vi "FrozenFraction_Calcualte.vi"(8 "FreezeIdx":i32[](array[numeric])=[255, 322, 264, 271, 213, 293, 124, 126, 128, 125, 124, 129, 98, 99, 102, 99, 98, 98, 0, 81, 76, 73, 80, 73, 242, 225, 335, 285, 302, 293, 131, 126, 127, 130, 129, 126, 100, 105, 106, 99, 98, 99, 0, 73, 75, 79, 77, 71, 272, 219, 231, 224, 285, 293, 130, 135, 124, 133, 126, 135, 98, 99, 108, 99, 99, 98, 0, 76, 75, 0, 77, 76, 236, 192, 232, 228, 284, 240, 125, 125, 126, 137, 128, 126, 105, 106, 96, 110, 99, 100, 71, 80, 77, 79, 74, 77, 335, 254, 302, 233, 271, 287, 128, 133, 136, 127, 128, 133, 99, 107, 100, 108, 101, 101, 80, 77, 76, 74, 73, 74, 287, 301, 265, 290, 280, 272, 128, 136, 130, 124, 123, 130, 102, 99, 108, 100, 107, 100, 76, 76, 82, 75, 73, 74, 303, 321, 285, 279, 243, 273, 126, 126, 125, 126, 132, 124, 98, 108, 104, 111, 99, 106, 84, 76, 75, 82, 89, 72, 320, 283, 291, 240, 297, 236, 129, 131, 129, 124, 131, 126, 100, 105, 99, 100, 99, 101, 81, 81, 75, 76, 77, 75, 243, 307, 301, 286, 267, 129, 124, 132, 125, 127, 125, 124, 97, 104, 100, 99, 100, 100, 0, 88, 76, 73, 75, 75, 209, 309, 219, 296, 262, 217, 127, 131, 134, 127, 127, 124, 104, 100, 108, 107, 98, 99, 0, 77, 83, 80, 71, 76, 191, 248, 312, 218, 143, 278, 126, 126, 131, 133, 125, 126, 97, 100, 98, 99, 104, 100, 0, 78, 81, 75, 76, 75, 311, 257, 192, 162, 147, 252, 126, 126, 126, 130, 124, 123, 98, 98, 97, 98, 98, 99, 74, 79, 72, 73, 74, 73, 316, 253, 172, 122, 302, 135, 129, 129, 130, 124, 136, 125, 99, 103, 97, 101, 98, 98, 77, 74, 74, 82, 74, 77, 234, 193, 182, 305, 170, 153, 126, 132, 125, 133, 126, 125, 99, 98, 99, 99, 99, 102, 72, 74, 73, 73, 74, 73, 271, 240, 181, 300, 248, 288, 124, 125, 133, 132, 129, 124, 97, 97, 98, 99, 99, 99, 78, 81, 74, 75, 75, 73, 238, 259, 221, 128, 214, 192, 128, 128, 128, 124, 126, 129, 99, 99, 98, 99, 98, 98, 75, 78, 74, 79, 73, 75], 9 "Temps":dbl[][](graph)=array384x528[202752 elements], 10 "FreezeTemps":dbl[](array[numeric])=[-17.28714285714284, -23.360476190476163, -18.044761904761884, -18.98333333333329, -13.286190476190427, -20.920476190476165, -5.292380952380938, -5.350476190476172, -5.453809523809525, -5.195714285714246, -5.249047619047587, -5.483333333333292, -2.8057142857142594, -2.902380952380952, -2.915714285714273, -2.8785714285713766, -2.9642857142857224, -3.019999999999982, 0.0, -1.2985714285713925, -0.7119047619047478, -0.5214285714285438, -0.0428571428570876, -0.5152380952380895, -16.166190476190422, -14.609999999999957, -25.292857142857116, -20.543333333333294, -22.113333333333287, -21.32571428571424, -5.505238095238042, -5.593809523809512, -5.405714285714225, -5.401428571428539, -5.500952380952356, -5.363333333333287, -3.08095238095234, -3.0838095238095207, -3.0514285714285734, -3.015714285714239, -2.96333333333331, -3.152380952380952, 0.0, -0.61761904761903, -0.7347619047618537, -0.5952380952380736, -0.6928571428571217, -0.4047619047618696, -19.03666666666666, -14.313333333333276, -15.039047619047608, -14.185238095238049, -20.61285714285711, -21.26190476190473, -5.579523809523778, -5.624285714285691, -5.4423809523809155, -5.434761904761899, -5.471904761904739, -5.935238095238049, -3.0038095238095366, -2.935714285714255, -2.964761904761872, -3.1223809523809223, -3.133333333333269, -2.9828571428570854, 0.0, -1.0409523809523193, -0.8623809523809314, 0.0, -0.1014285714285847, -0.7966666666666242, -15.671428571428578, -11.62428571428569, -15.217142857142846, -14.780476190476179, -20.487619047619006, -16.03047619047618, -5.399523809523771, -5.3642857142857, -5.5033333333332735, -5.954285714285675, -5.610476190476163, -5.480476190476168, -3.2566666666666606, -3.0785714285713652, -2.83428571428567, -3.031904761904741, -3.0571428571428214, -3.1619047619047365, -0.6461904761904407, -1.014285714285677, -0.8404761904761813, -0.9290476190475943, -0.8390476190476193, -0.8742857142856906, -25.16952380952378, -17.619999999999976, -22.054285714285697, -14.887142857142862, -19.3942857142857, -20.490952380952336, -5.6619047619047365, -5.628571428571377, -5.825714285714241, -5.541904761904732, -5.704761904761881, -5.809523809523796, -3.402380952380952, -3.1676190476190413, -3.2052380952380872, -3.1780952380951817, -3.08428571428567, -3.1638095238095048, -1.1566666666666379, -0.8852380952380372, -0.9509523809523444, -0.784761904761865, -0.6295238095237892, -0.5247619047618741, -20.52047619047616, -22.020952380952338, -18.561428571428564, -21.041904761904732, -20.22999999999996, -19.46857142857138, -5.632380952380913, -5.829047619047628, -5.757619047619016, -5.409999999999968, -5.2971428571428305, -5.7942857142857065, -3.439047619047585, -3.210476190476129, -3.2157142857142276, -3.1152380952380554, -3.0599999999999454, -2.903809523809514, -0.9961904761904066, -1.029047619047617, -0.9152380952380668, -0.8190476190475806, -0.4390476190475852, -0.7114285714285415, -21.997619047619025, -23.774285714285696, -20.46666666666664, -19.79761904761901, -16.629999999999995, -19.37476190476187, -5.673809523809496, -5.544761904761856, -5.559523809523796, -5.588571428571413, -5.5719047619047615, -5.441904761904766, -3.299047619047599, -3.1723809523809336, -3.216190476190434, -3.300476190476161, -2.9395238095237914, -3.2376190476190345, -1.2780952380952044, -0.9566666666666492, -1.0123809523809086, -0.4071428571428441, -0.1261904761904589, -0.6047619047618582, -23.76714285714283, -20.47142857142856, -20.978095238095193, -16.091904761904743, -22.034285714285687, -16.039999999999964, -5.609047619047601, -5.653333333333308, -5.613333333333287, -5.550476190476161, -5.621904761904716, -5.621904761904716, -3.3133333333332757, -3.3828571428571195, -3.167142857142835, -3.2052380952380872, -3.2128571428571036, -3.1499999999999773, -1.1733333333332894, -1.3190476190475806, -0.8604761904761631, -1.011428571428553, -0.9661904761904339, -0.8266666666666538, -16.467142857142846, -22.642380952380933, -21.78380952380951, -20.803333333333285, -18.689047619047614, -5.77571428571423, -5.7071428571428555, -5.840952380952331, -5.715238095238078, -5.647619047619003, -5.512380952380909, -5.458095238095211, -3.29047619047617, -3.388095238095218, -3.332857142857108, -3.2142857142857224, -3.185714285714255, -3.296190476190418, 0.0, -1.360476190476163, -0.9638095238095161, -0.7519047619047683, -0.8533333333332962, -0.7152380952380781, -13.07714285714286, -22.502857142857096, -14.274285714285725, -21.791904761904732, -18.57238095238094, -14.203809523809525, -5.652380952380952, -5.71666666666664, -5.596666666666636, -5.579047619047628, -5.486666666666679, -5.535714285714221, -3.5138095238095275, -3.322857142857117, -3.3861904761904498, -3.308095238095177, -3.056666666666672, -3.133333333333269, 0.0, -1.0552380952380531, -0.9566666666666492, -0.8438095238095116, -0.5733333333332666, -0.8880952380952181, -11.63952380952378, -16.895714285714234, -23.103333333333296, -14.486666666666679, -6.6823809523809246, -19.833333333333286, -5.862857142857138, -5.714761904761872, -5.702857142857113, -5.740952380952365, -5.64285714285711, -5.604285714285709, -3.1357142857142435, -3.3133333333332757, -3.1299999999999955, -3.1995238095237823, -3.238095238095184, -3.1633333333332985, 0.0, -0.9942857142856951, -0.9276190476190322, -0.8047619047619037, -0.8871428571428623, -0.9176190476190413, -22.81761904761902, -17.840476190476153, -11.563809523809539, -8.832857142857108, -7.065238095238044, -17.505714285714248, -5.720952380952326, -5.677619047619032, -5.690476190476147, -5.643809523809523, -5.464761904761872, -5.563333333333276, -3.345714285714223, -3.254285714285686, -2.8928571428571104, -3.0804761904761335, -2.969523809523764, -3.0995238095238165, -1.1228571428571286, -0.9161904761904225, -0.6747619047619082, -0.781904761904741, -0.8728571428571286, -0.6352380952380372, -23.009999999999962, -17.229523809523783, -9.71999999999997, -5.177142857142826, -22.008095238095194, -5.899999999999977, -5.7390476190475965, -5.714285714285722, -5.618095238095179, -5.594761904761867, -5.941904761904766, -5.534285714285716, -3.293333333333294, -3.2347619047618537, -2.966190476190434, -3.1838095238094866, -2.9609523809523353, -3.0385714285714016, -1.167142857142835, -1.0023809523809177, -0.9547619047618809, -0.9495238095237823, -0.8280952380952158, -0.8585714285713948, -15.54095238095232, -11.46999999999997, -10.558095238095177, -22.105714285714242, -9.649523809523771, -8.017142857142858, -5.544761904761856, -5.662380952380943, -5.586190476190438, -5.632380952380913, -5.582380952380902, -5.65476190476187, -3.2333333333332916, -3.0485714285713925, -3.2085714285713607, -3.1385714285713675, -3.2114285714285415, -3.283333333333303, -0.5752380952380918, -0.8571428571428328, -0.7447619047619014, -0.6280952380952272, -0.8199999999999932, -0.6380952380952181, -18.772857142857106, -16.079523809523778, -10.479523809523812, -21.853333333333296, -16.9080952380952, -20.799523809523777, -5.465714285714228, -5.371904761904716, -5.692857142857122, -5.553809523809491, -5.554761904761904, -5.547619047619037, -2.9614285714285415, -2.967619047618996, -3.189047619047585, -3.2057142857142367, -2.995238095238051, -3.0338095238095093, -1.1819047619047183, -0.7414285714285711, -0.8514285714285847, -0.6380952380952181, -0.6257142857142526, -0.5314285714285347, -15.450476190476138, -17.551428571428545, -14.244285714285695, -5.428095238095182, -13.503809523809537, -11.372380952380922, -5.407142857142844, -5.306190476190409, -5.479999999999961, -5.233333333333292, -5.076666666666654, -5.421428571428578, -2.956190476190443, -2.809523809523796, -2.8680952380951794, -2.8466666666666356, -2.704761904761881, -2.7071428571428555, -0.3071428571428214, -0.5847619047618764, -0.5171428571428578, -0.3957142857142344, -0.4861904761904157, -0.4599999999999795], 11 "PartitionArray":string[](array[string])=["A, MQ unfiltered", "A, MQ unfiltered", "A, MQ unfiltered", "B, D2O unfiltered", "B, D2O unfiltered", "B, D2O unfiltered", "C, 1mg/ml Snomax in MQ", "C, 1mg/ml Snomax in MQ", "C, 1mg/ml Snomax in MQ", "C, 1mg/ml Snomax in MQ", "C, 1mg/ml Snomax in MQ", "C, 1mg/ml Snomax in MQ", "D, 1mg/ml Snomax in 1:1 MQ:D2O", "D, 1mg/ml Snomax in 1:1 MQ:D2O", "D, 1mg/ml Snomax in 1:1 MQ:D2O", "D, 1mg/ml Snomax in 1:1 MQ:D2O", "D, 1mg/ml Snomax in 1:1 MQ:D2O", "D, 1mg/ml Snomax in 1:1 MQ:D2O", "E, 1mg/ml Snomax in D2O", "E, 1mg/ml Snomax in D2O", "E, 1mg/ml Snomax in D2O", "E, 1mg/ml Snomax in D2O", "E, 1mg/ml Snomax in D2O", "E, 1mg/ml Snomax in D2O", "A, MQ unfiltered", "A, MQ unfiltered", "A, MQ unfiltered", "B, D2O unfiltered", "B, D2O unfiltered", "B, D2O unfiltered", "C, 1mg/ml Snomax in MQ", "C, 1mg/ml Snomax in MQ", "C, 1mg/ml Snomax in MQ", "C, 1mg/ml Snomax in MQ", "C, 1mg/ml Snomax in MQ", "C, 1mg/ml Snomax in MQ", "D, 1mg/ml Snomax in 1:1 MQ:D2O", "D, 1mg/ml Snomax in 1:1 MQ:D2O", "D, 1mg/ml Snomax in 1:1 MQ:D2O", "D, 1mg/ml Snomax in 1:1 MQ:D2O", "D, 1mg/ml Snomax in 1:1 MQ:D2O", "D, 1mg/ml Snomax in 1:1 MQ:D2O", "E, 1mg/ml Snomax in D2O", "E, 1mg/ml Snomax in D2O", "E, 1mg/ml Snomax in D2O", "E, 1mg/ml Snomax in D2O", "E, 1mg/ml Snomax in D2O", "E, 1mg/ml Snomax in D2O", "A, MQ unfiltered", "A, MQ unfiltered", "A, MQ unfiltered", "B, D2O unfiltered", "B, D2O unfiltered", "B, D2O unfiltered", "C, 1mg/ml Snomax in MQ", "C, 1mg/ml Snomax in MQ", "C, 1mg/ml Snomax in MQ", "C, 1mg/ml Snomax in MQ", "C, 1mg/ml Snomax in MQ", "C, 1mg/ml Snomax in MQ", "D, 1mg/ml Snomax in 1:1 MQ:D2O", "D, 1mg/ml Snomax in 1:1 MQ:D2O", "D, 1mg/ml Snomax in 1:1 MQ:D2O", "D, 1mg/ml Snomax in 1:1 MQ:D2O", "D, 1mg/ml Snomax in 1:1 MQ:D2O", "D, 1mg/ml Snomax in 1:1 MQ:D2O", "E, 1mg/ml Snomax in D2O", "E, 1mg/ml Snomax in D2O", "E, 1mg/ml Snomax in D2O", "E, 1mg/ml Snomax in D2O", "E, 1mg/ml Snomax in D2O", "E, 1mg/ml Snomax in D2O", "A, MQ unfiltered", "A, MQ unfiltered", "A, MQ unfiltered", "B, D2O unfiltered", "B, D2O unfiltered", "B, D2O unfiltered", "C, 1mg/ml Snomax in MQ", "C, 1mg/ml Snomax in MQ", "C, 1mg/ml Snomax in MQ", "C, 1mg/ml Snomax in MQ", "C, 1mg/ml Snomax in MQ", "C, 1mg/ml Snomax in MQ", "D, 1mg/ml Snomax in 1:1 MQ:D2O", "D, 1mg/ml Snomax in 1:1 MQ:D2O", "D, 1mg/ml Snomax in 1:1 MQ:D2O", "D, 1mg/ml Snomax in 1:1 MQ:D2O", "D, 1mg/ml Snomax in 1:1 MQ:D2O", "D, 1mg/ml Snomax in 1:1 MQ:D2O", "E, 1mg/ml Snomax in D2O", "E, 1mg/ml Snomax in D2O", "E, 1mg/ml Snomax in D2O", "E, 1mg/ml Snomax in D2O", "E, 1mg/ml Snomax in D2O", "E, 1mg/ml Snomax in D2O", "A, MQ unfiltered", "A, MQ unfiltered", "A, MQ unfiltered", "B, D2O unfiltered", "B, D2O unfiltered", "B, D2O unfiltered", "C, 1mg/ml Snomax in MQ", "C, 1mg/ml Snomax in MQ", "C, 1mg/ml Snomax in MQ", "C, 1mg/ml Snomax in MQ", "C, 1mg/ml Snomax in MQ", "C, 1mg/ml Snomax in MQ", "D, 1mg/ml Snomax in 1:1 MQ:D2O", "D, 1mg/ml Snomax in 1:1 MQ:D2O", "D, 1mg/ml Snomax in 1:1 MQ:D2O", "D, 1mg/ml Snomax in 1:1 MQ:D2O", "D, 1mg/ml Snomax in 1:1 MQ:D2O", "D, 1mg/ml Snomax in 1:1 MQ:D2O", "E, 1mg/ml Snomax in D2O", "E, 1mg/ml Snomax in D2O", "E, 1mg/ml Snomax in D2O", "E, 1mg/ml Snomax in D2O", "E, 1mg/ml Snomax in D2O", "E, 1mg/ml Snomax in D2O", "A, MQ unfiltered", "A, MQ unfiltered", "A, MQ unfiltered", "B, D2O unfiltered", "B, D2O unfiltered", "B, D2O unfiltered", "C, 1mg/ml Snomax in MQ", "C, 1mg/ml Snomax in MQ", "C, 1mg/ml Snomax in MQ", "C, 1mg/ml Snomax in MQ", "C, 1mg/ml Snomax in MQ", "C, 1mg/ml Snomax in MQ", "D, 1mg/ml Snomax in 1:1 MQ:D2O", "D, 1mg/ml Snomax in 1:1 MQ:D2O", "D, 1mg/ml Snomax in 1:1 MQ:D2O", "D, 1mg/ml Snomax in 1:1 MQ:D2O", "D, 1mg/ml Snomax in 1:1 MQ:D2O", "D, 1mg/ml Snomax in 1:1 MQ:D2O", "E, 1mg/ml Snomax in D2O", "E, 1mg/ml Snomax in D2O", "E, 1mg/ml Snomax in D2O", "E, 1mg/ml Snomax in D2O", "E, 1mg/ml Snomax in D2O", "E, 1mg/ml Snomax in D2O", "A, MQ unfiltered", "A, MQ unfiltered", "A, MQ unfiltered", "B, D2O unfiltered", "B, D2O unfiltered", "B, D2O unfiltered", "C, 1mg/ml Snomax in MQ", "C, 1mg/ml Snomax in MQ", "C, 1mg/ml Snomax in MQ", "C, 1mg/ml Snomax in MQ", "C, 1mg/ml Snomax in MQ", "C, 1mg/ml Snomax in MQ", "D, 1mg/ml Snomax in 1:1 MQ:D2O", "D, 1mg/ml Snomax in 1:1 MQ:D2O", "D, 1mg/ml Snomax in 1:1 MQ:D2O", "D, 1mg/ml Snomax in 1:1 MQ:D2O", "D, 1mg/ml Snomax in 1:1 MQ:D2O", "D, 1mg/ml Snomax in 1:1 MQ:D2O", "E, 1mg/ml Snomax in D2O", "E, 1mg/ml Snomax in D2O", "E, 1mg/ml Snomax in D2O", "E, 1mg/ml Snomax in D2O", "E, 1mg/ml Snomax in D2O", "E, 1mg/ml Snomax in D2O", "A, MQ unfiltered", "A, MQ unfiltered", "A, MQ unfiltered", "B, D2O unfiltered", "B, D2O unfiltered", "B, D2O unfiltered", "C, 1mg/ml Snomax in MQ", "C, 1mg/ml Snomax in MQ", "C, 1mg/ml Snomax in MQ", "C, 1mg/ml Snomax in MQ", "C, 1mg/ml Snomax in MQ", "C, 1mg/ml Snomax in MQ", "D, 1mg/ml Snomax in 1:1 MQ:D2O", "D, 1mg/ml Snomax in 1:1 MQ:D2O", "D, 1mg/ml Snomax in 1:1 MQ:D2O", "D, 1mg/ml Snomax in 1:1 MQ:D2O", "D, 1mg/ml Snomax in 1:1 MQ:D2O", "D, 1mg/ml Snomax in 1:1 MQ:D2O", "E, 1mg/ml Snomax in D2O", "E, 1mg/ml Snomax in D2O", "E, 1mg/ml Snomax in D2O", "E, 1mg/ml Snomax in D2O", "E, 1mg/ml Snomax in D2O", "E, 1mg/ml Snomax in D2O", "A, MQ unfiltered", "A, MQ unfiltered", "A, MQ unfiltered", "B, D2O unfiltered", "B, D2O unfiltered", "B, D2O unfiltered", "C, 1mg/ml Snomax in MQ", "C, 1mg/ml Snomax in MQ", "C, 1mg/ml Snomax in MQ", "C, 1mg/ml Snomax in MQ", "C, 1mg/ml Snomax in MQ", "C, 1mg/ml Snomax in MQ", "D, 1mg/ml Snomax in 1:1 MQ:D2O", "D, 1mg/ml Snomax in 1:1 MQ:D2O", "D, 1mg/ml Snomax in 1:1 MQ:D2O", "D, 1mg/ml Snomax in 1:1 MQ:D2O", "D, 1mg/ml Snomax in 1:1 MQ:D2O", "D, 1mg/ml Snomax in 1:1 MQ:D2O", "E, 1mg/ml Snomax in D2O", "E, 1mg/ml Snomax in D2O", "E, 1mg/ml Snomax in D2O", "E, 1mg/ml Snomax in D2O", "E, 1mg/ml Snomax in D2O", "E, 1mg/ml Snomax in D2O", "A, MQ unfiltered", "A, MQ unfiltered", "A, MQ unfiltered", "B, D2O unfiltered", "B, D2O unfiltered", "B, D2O unfiltered", "C, 1mg/ml Snomax in MQ", "C, 1mg/ml Snomax in MQ", "C, 1mg/ml Snomax in MQ", "C, 1mg/ml Snomax in MQ", "C, 1mg/ml Snomax in MQ", "C, 1mg/ml Snomax in MQ", "D, 1mg/ml Snomax in 1:1 MQ:D2O", "D, 1mg/ml Snomax in 1:1 MQ:D2O", "D, 1mg/ml Snomax in 1:1 MQ:D2O", "D, 1mg/ml Snomax in 1:1 MQ:D2O", "D, 1mg/ml Snomax in 1:1 MQ:D2O", "D, 1mg/ml Snomax in 1:1 MQ:D2O", "E, 1mg/ml Snomax in D2O", "E, 1mg/ml Snomax in D2O", "E, 1mg/ml Snomax in D2O", "E, 1mg/ml Snomax in D2O", "E, 1mg/ml Snomax in D2O", "E, 1mg/ml Snomax in D2O", "A, MQ unfiltered", "A, MQ unfiltered", "A, MQ unfiltered", "B, D2O unfiltered", "B, D2O unfiltered", "B, D2O unfiltered", "C, 1mg/ml Snomax in MQ", "C, 1mg/ml Snomax in MQ", "C, 1mg/ml Snomax in MQ", "C, 1mg/ml Snomax in MQ", "C, 1mg/ml Snomax in MQ", "C, 1mg/ml Snomax in MQ", "D, 1mg/ml Snomax in 1:1 MQ:D2O", "D, 1mg/ml Snomax in 1:1 MQ:D2O", "D, 1mg/ml Snomax in 1:1 MQ:D2O", "D, 1mg/ml Snomax in 1:1 MQ:D2O", "D, 1mg/ml Snomax in 1:1 MQ:D2O", "D, 1mg/ml Snomax in 1:1 MQ:D2O", "E, 1mg/ml Snomax in D2O", "E, 1mg/ml Snomax in D2O", "E, 1mg/ml Snomax in D2O", "E, 1mg/ml Snomax in D2O", "E, 1mg/ml Snomax in D2O", "E, 1mg/ml Snomax in D2O", "A, MQ unfiltered", "A, MQ unfiltered", "A, MQ unfiltered", "B, D2O unfiltered", "B, D2O unfiltered", "B, D2O unfiltered", "C, 1mg/ml Snomax in MQ", "C, 1mg/ml Snomax in MQ", "C, 1mg/ml Snomax in MQ", "C, 1mg/ml Snomax in MQ", "C, 1mg/ml Snomax in MQ", "C, 1mg/ml Snomax in MQ", "D, 1mg/ml Snomax in 1:1 MQ:D2O", "D, 1mg/ml Snomax in 1:1 MQ:D2O", "D, 1mg/ml Snomax in 1:1 MQ:D2O", "D, 1mg/ml Snomax in 1:1 MQ:D2O", "D, 1mg/ml Snomax in 1:1 MQ:D2O", "D, 1mg/ml Snomax in 1:1 MQ:D2O", "E, 1mg/ml Snomax in D2O", "E, 1mg/ml Snomax in D2O", "E, 1mg/ml Snomax in D2O", "E, 1mg/ml Snomax in D2O", "E, 1mg/ml Snomax in D2O", "E, 1mg/ml Snomax in D2O", "A, MQ unfiltered", "A, MQ unfiltered", "A, MQ unfiltered", "B, D2O unfiltered", "B, D2O unfiltered", "B, D2O unfiltered", "C, 1mg/ml Snomax in MQ", "C, 1mg/ml Snomax in MQ", "C, 1mg/ml Snomax in MQ", "C, 1mg/ml Snomax in MQ", "C, 1mg/ml Snomax in MQ", "C, 1mg/ml Snomax in MQ", "D, 1mg/ml Snomax in 1:1 MQ:D2O", "D, 1mg/ml Snomax in 1:1 MQ:D2O", "D, 1mg/ml Snomax in 1:1 MQ:D2O", "D, 1mg/ml Snomax in 1:1 MQ:D2O", "D, 1mg/ml Snomax in 1:1 MQ:D2O", "D, 1mg/ml Snomax in 1:1 MQ:D2O", "E, 1mg/ml Snomax in D2O", "E, 1mg/ml Snomax in D2O", "E, 1mg/ml Snomax in D2O", "E, 1mg/ml Snomax in D2O", "E, 1mg/ml Snomax in D2O", "E, 1mg/ml Snomax in D2O", "A, MQ unfiltered", "A, MQ unfiltered", "A, MQ unfiltered", "B, D2O unfiltered", "B, D2O unfiltered", "B, D2O unfiltered", "C, 1mg/ml Snomax in MQ", "C, 1mg/ml Snomax in MQ", "C, 1mg/ml Snomax in MQ", "C, 1mg/ml Snomax in MQ", "C, 1mg/ml Snomax in MQ", "C, 1mg/ml Snomax in MQ", "D, 1mg/ml Snomax in 1:1 MQ:D2O", "D, 1mg/ml Snomax in 1:1 MQ:D2O", "D, 1mg/ml Snomax in 1:1 MQ:D2O", "D, 1mg/ml Snomax in 1:1 MQ:D2O", "D, 1mg/ml Snomax in 1:1 MQ:D2O", "D, 1mg/ml Snomax in 1:1 MQ:D2O", "E, 1mg/ml Snomax in D2O", "E, 1mg/ml Snomax in D2O", "E, 1mg/ml Snomax in D2O", "E, 1mg/ml Snomax in D2O", "E, 1mg/ml Snomax in D2O", "E, 1mg/ml Snomax in D2O", "A, MQ unfiltered", "A, MQ unfiltered", "A, MQ unfiltered", "B, D2O unfiltered", "B, D2O unfiltered", "B, D2O unfiltered", "C, 1mg/ml Snomax in MQ", "C, 1mg/ml Snomax in MQ", "C, 1mg/ml Snomax in MQ", "C, 1mg/ml Snomax in MQ", "C, 1mg/ml Snomax in MQ", "C, 1mg/ml Snomax in MQ", "D, 1mg/ml Snomax in 1:1 MQ:D2O", "D, 1mg/ml Snomax in 1:1 MQ:D2O", "D, 1mg/ml Snomax in 1:1 MQ:D2O", "D, 1mg/ml Snomax in 1:1 MQ:D2O", "D, 1mg/ml Snomax in 1:1 MQ:D2O", "D, 1mg/ml Snomax in 1:1 MQ:D2O", "E, 1mg/ml Snomax in D2O", "E, 1mg/ml Snomax in D2O", "E, 1mg/ml Snomax in D2O", "E, 1mg/ml Snomax in D2O", "E, 1mg/ml Snomax in D2O", "E, 1mg/ml Snomax in D2O", "A, MQ unfiltered", "A, MQ unfiltered", "A, MQ unfiltered", "B, D2O unfiltered", "B, D2O unfiltered", "B, D2O unfiltered", "C, 1mg/ml Snomax in MQ", "C, 1mg/ml Snomax in MQ", "C, 1mg/ml Snomax in MQ", "C, 1mg/ml Snomax in MQ", "C, 1mg/ml Snomax in MQ", "C, 1mg/ml Snomax in MQ", "D, 1mg/ml Snomax in 1:1 MQ:D2O", "D, 1mg/ml Snomax in 1:1 MQ:D2O", "D, 1mg/ml Snomax in 1:1 MQ:D2O", "D, 1mg/ml Snomax in 1:1 MQ:D2O", "D, 1mg/ml Snomax in 1:1 MQ:D2O", "D, 1mg/ml Snomax in 1:1 MQ:D2O", "E, 1mg/ml Snomax in D2O", "E, 1mg/ml Snomax in D2O", "E, 1mg/ml Snomax in D2O", "E, 1mg/ml Snomax in D2O", "E, 1mg/ml Snomax in D2O", "E, 1mg/ml Snomax in D2O"]) -> (2 "FreezeFract Concatinated":dbl[](array[numeric]), 3 "FrozenFractionGraph":dbl[][](graph))   [LabVIEW 2020]
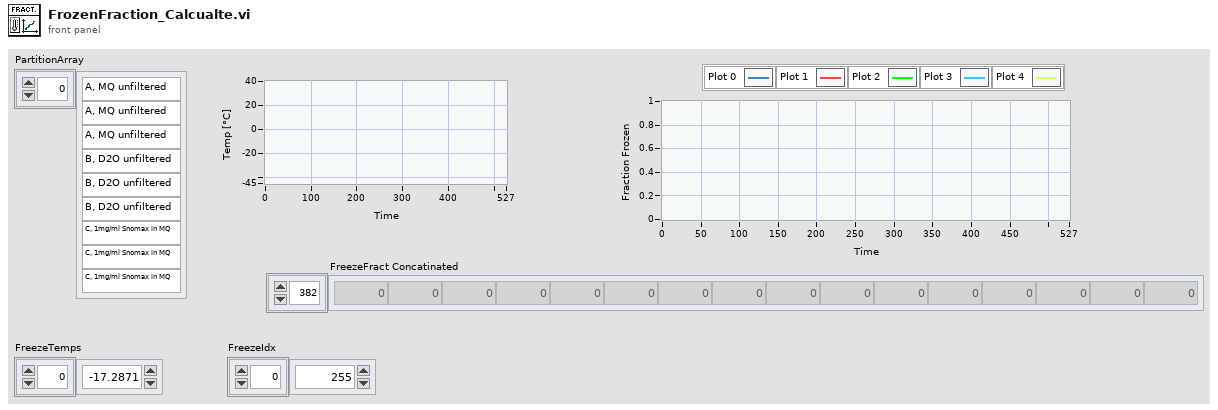
[diagram p1: front panel]
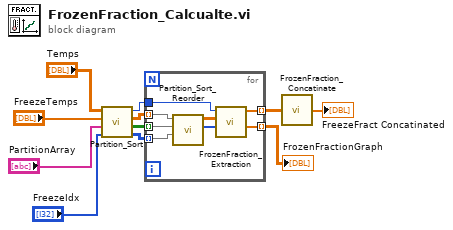
[diagram p0: block diagram]
diagram:
  n1 = call "Partition_Sort.vi"("FreezeIdx"="FreezeIdx", "PartitionArray"="PartitionArray", "FreezeTemps"="FreezeTemps", "Temps"="Temps") -> ("Freeze Idx / Part Array"=w2:i32[][], "Freeze / Part Array"=w9:bool[][], "FreezeTenos / Part Array"=w10:dbl[][], "MaxSize"=w3:i32)  [unwired: 4 in]
  n2 = for {
    tunnel: w10 -> [w19] mode=indexing
    tunnel: [w16] -> w7 mode=indexing
    tunnel: w9 -> [w17] mode=indexing
    tunnel: w2 -> [w15] mode=indexing
    tunnel: [w14] -> w4 mode=indexing
    tunnel: w3 -> [w12]
    n3 = call "Partition_Sort_Reorder.vi"("Freeze Idx / Part Array"=w15, "Freeze / Part Array"=w17, "FreezeTemps / Part Array"=w19) -> ("Sorted Freeze Idx / Part > idx"=w13:i32[], "Sorted Freeze / Part > idx"=w18:dbl[][])  [unwired: 7 in]
    n4 = call "FrozenFraction_Extraction.vi"("Sorted Freeze Idx / Part > idx"=w13, "Sorted Freeze / Part > idx"=w18, "MaxSize"=w12) -> ("FroozenFraction Graph"=w14:dbl[], "Freeze Fraction"=w16:dbl[])  [unwired: 7 in]
  }
  "FrozenFractionGraph" <- w4
  n5 = call "FrozenFraction_Concatinate.vi"("Freeze Fraction"=w7) -> ("Freeze Fraction Concatinated"=→"FreezeFract Concatinated":dbl[])
